vi "ForceIdleGLOBAL (1).vi"() -> ()   [LabVIEW 2017]
panel:
  out "ForceIdleGlobal":bool
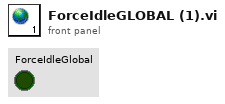
[diagram p1: front panel]
diagram:
